vi "Open log.vi"() -> ()   [LabVIEW 2015]
uses:
  Shared/Types/Compiled Data.ctl
  Shared/Types/RT Init Data.ctl
  Shared/Types/RT Status.ctl
  Shared/Types/9759 RevB.ctl
  NI 9759 RevB Custom Device.lvlib
panel:
  out "Compiled Data":T1 {"9759 RevB"."Settings"."ControlCals"."ThetaLH (deg)" format="%.3f"; "9759 RevB"."Settings"."ControlCals"."ULHLag (sec)" format="%.3f"; "9759 RevB"."Settings"."ControlCals"."USLag (sec)" format="%.3f"; "9759 RevB"."Settings"."ControlCals"."TLead (sec)" format="%.3f"; "9759 RevB"."Settings"."ControlCals"."TLag (sec)" format="%.3f"}
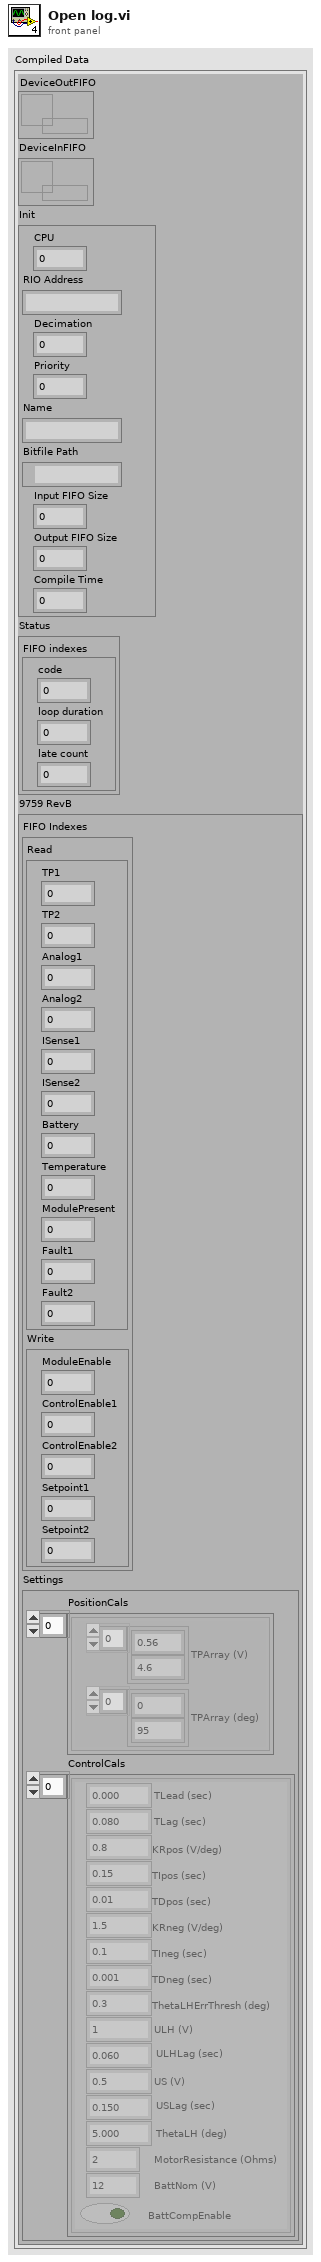
[diagram p1: front panel]
types:
  T1 = typedef "NI 9759 RevB Custom Device.lvlib/Compiled Data.ctl" = cluster{"DeviceOutFIFO":refnum<k33>, "DeviceInFIFO":refnum<k33>, "Init":T2, "Status":T3, "9759 RevB":T4}
  T2 = typedef "NI 9759 RevB Custom Device.lvlib/RT Init Data.ctl" = cluster{"CPU":i32, "RIO Address":string, "Decimation":i32, "Priority":i32, "Name":string, "Bitfile Path":path, "Input FIFO Size":i32, "Output FIFO Size":i32, "Compile Time":dbl}
  T3 = typedef "NI 9759 RevB Custom Device.lvlib/RT Status.ctl" = cluster{"FIFO indexes":cluster{"code":i32, "loop duration":i32, "late count":i32}}
  T4 = typedef "NI 9759 RevB Custom Device.lvlib/9759 RevB.ctl" = cluster{"FIFO Indexes":cluster{"Read":cluster{"TP1":i32, "TP2":i32, "Analog1":i32, "Analog2":i32, "ISense1":i32, "ISense2":i32, "Battery":i32, "Temperature":i32, "ModulePresent":i32, "Fault1":i32, "Fault2":i32}, "Write":cluster{"ModuleEnable":i32, "ControlEnable1":i32, "ControlEnable2":i32, "Setpoint1":i32, "Setpoint2":i32}}, "Settings":cluster{"PositionCals":cluster{"TPArray (V)":sgl[], "TPArray (deg)":sgl[]}[], "ControlCals":cluster{"TLead (sec)":sgl, "TLag (sec)":sgl, "KRpos (V/deg)":sgl, "TIpos (sec)":sgl, "TDpos (sec)":sgl, "KRneg (V/deg)":sgl, "TIneg (sec)":sgl, "TDneg (sec)":sgl, "ThetaLHErrThresh (deg)":sgl, "ULH (V)":sgl, "ULHLag (sec)":sgl, "US (V)":sgl, "USLag (sec)":sgl, "ThetaLH (deg)":sgl, "MotorResistance (Ohms)":sgl, "BattNom (V)":sgl, "BattCompEnable":bool}[]}}
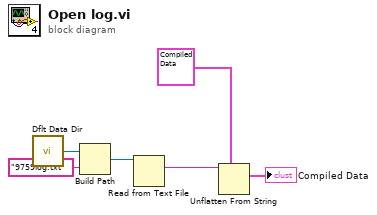
[diagram p0: block diagram]
diagram:
  n1 = call <vilib>:"Dflt Data Dir.vi"() -> ("App:Default Data Directory"=w3:path)
  n2 = Build Path(base path=w3, name or relative path="9759log.txt") -> (appended path=w1:path)
  n3 = Read from Text File(file (use dialog)=w1) -> (text=w6:string)  [unwired: 3 in, 3 out]
  n4 = Unflatten From String(type=T1 {"DeviceOutFIFO"=refnum, "DeviceInFIFO"=refnum, "Init"={"CPU"=0, "RIO Address"="", "Decimation"=0, "Priority"=0, "Name"="", "Bitfile Path"=path "", "Input FIFO Size"=0, "Output FIFO Size"=0, "Compile Time"=0.0}, "Status"={"FIFO indexes"={"code"=0, "loop duration"=0, "late count"=0}}, "9759 RevB"={"FIFO Indexes"={"Read"={"TP1"=0, "TP2"=0, "Analog1"=0, "Analog2"=0, "ISense1"=0, "ISense2"=0, "Battery"=0, "Temperature"=0, "ModulePresent"=0, "Fault1"=0, "Fault2"=0}, "Write"={"ModuleEnable"=0, "ControlEnable1"=0, "ControlEnable2"=0, "Setpoint1"=0, "Setpoint2"=0}}, "Settings"={"PositionCals"=[], "ControlCals"=[]}}} ("Compiled Data"), binary string=w6) -> (value=→"Compiled Data":T1)  [unwired: 3 in, 2 out]
